vi "Injector Settings FG.vi"(6 "Action":enum8{"GET", "SET"}(ring), 8 "error in (no error)":errorcluster, 10 "Fuel Injector settings":T1={"Name"="", "Channel index"=0, "Injector Refs"={"RunTimeSettings VS Ch Refs "=18446744073709551615, "Results VS Ch Refs"=18446744073709551615, "Voltage Wfm Ref"=0, "Current Wfm Ref"=0}} {"Injector Refs"."Results VS Ch Refs" format="%.0x"; "Injector Refs"."RunTimeSettings VS Ch Refs" format="%.0x"}, 11 "Item Ref":T2 format="%.0x") -> (0 "error out":errorcluster, 2 "Fuel Injector settings":T1={"Name"="", "Channel index"=0, "Injector Refs"={"RunTimeSettings VS Ch Refs "=18446744073709551615, "Results VS Ch Refs"=18446744073709551615, "Voltage Wfm Ref"=0, "Current Wfm Ref"=0}} {"Injector Refs"."Results VS Ch Refs" format="%.0x"; "Injector Refs"."RunTimeSettings VS Ch Refs" format="%.0x"}, 3 "Item Ref out":T2=18446744073709551615 format="%.0x")   [LabVIEW 2015]
uses:
  <vilib>/NI VeriStand/Custom Device API/Custom Device API.lvlib
  <vilib>/NI Veristand/Custom Device API/Get Item Property (Path).vi
  <vilib>/NI Veristand/Custom Device API/Custom Device Item Ref.ctl
  <vilib>/NI Veristand/Custom Device API/Waveform Data Reference.ctl
  Fuel Injector Settings.ctl
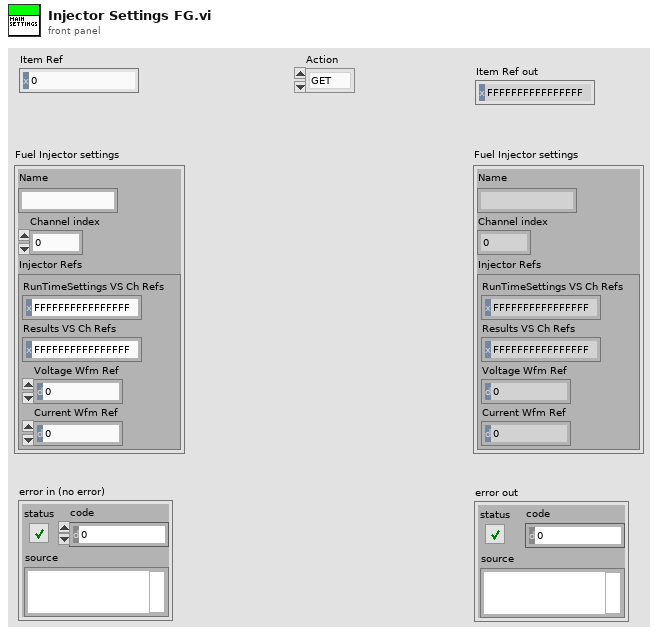
[diagram p1: front panel]
types:
  T1 = typedef "Fuel Injector Settings.ctl" = cluster{"Name":string, "Channel index":u16, "Injector Refs":cluster{"RunTimeSettings VS Ch Refs ":T2, "Results VS Ch Refs":T2, "Voltage Wfm Ref":T3, "Current Wfm Ref":T3}}
  T2 = typedef "Custom Device API.lvlib/Custom Device Item Ref.ctl" = u64
  T3 = typedef "Custom Device API.lvlib/Waveform Data Reference.ctl" = i32
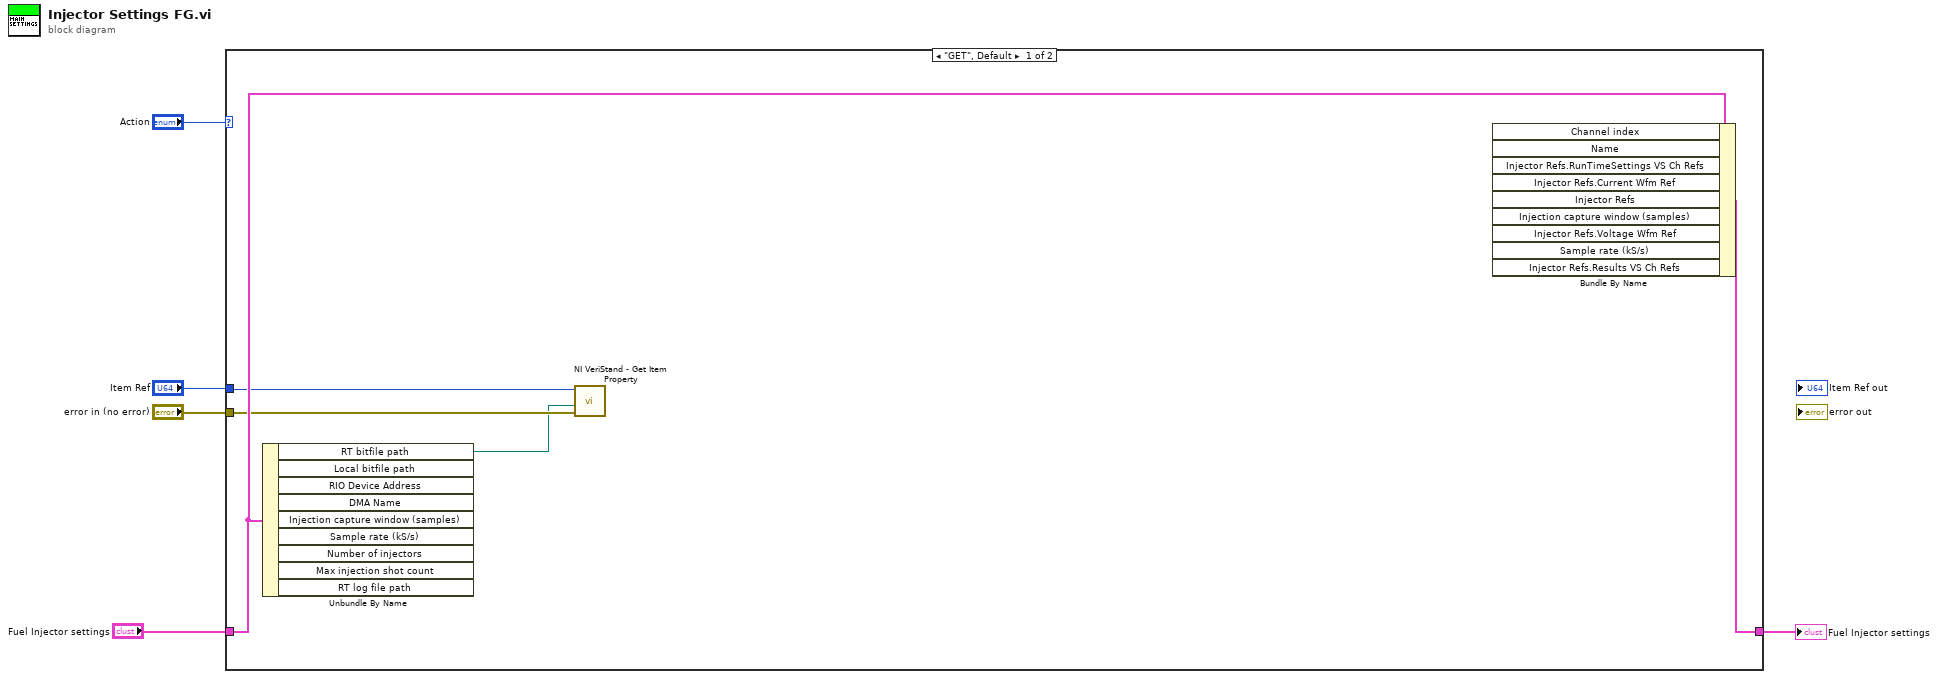
[diagram p0: block diagram]
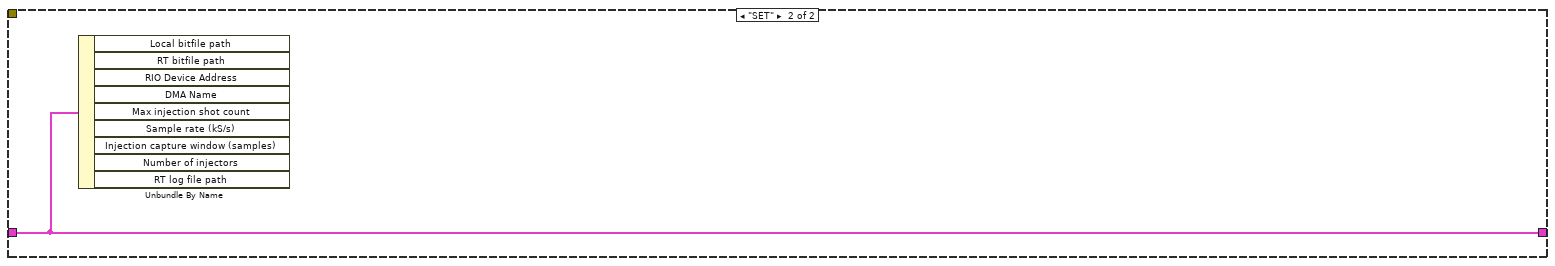
[diagram p2: hidden frame]
diagram:
  n1 = case shown="\"GET\", Default" "Action" {
    tunnel: "error in (no error)" -> [w7 _]
    tunnel: "Item Ref" -> [w8 _]
    tunnel: "Fuel Injector settings" -> [w10 w11]
    tunnel: [w9 w11] -> w1
    frame "GET", Default {
      n2 = Unbundle By Name(w10) -> ("RT bitfile path"=w6:path)  [unwired: 8 out]
      n3 = call-poly <vilib>:"NI VeriStand - Get Item Property.vi"("error in (no error)"=w7, "Default Value"=w6, "Item Ref in"=w8) -> ()  [unwired: 5 in, 4 out]
      n4 = Bundle By Name(cluster=w10) -> (w9:T1)  [unwired: 9 in]
    }
    frame "SET" {
      n5 = Unbundle By Name(w11) -> ()  [unwired: 9 out]
    }
  }
  "Fuel Injector settings" <- w1
